vi "AudioTest.Config - Read Plot Analysis Params.vi"(11 "Config Dir":path=path "C:/MTE/Audio Test/Config") -> (1 "Avg(F)/Float(T)":bool, 2 "End Freq":dbl=20000.0, 3 "Start Freq":dbl=500.0)   [LabVIEW 2018]
uses:
  <vilib>/Utility/config.llb/Read Key (Boolean).vi
  <vilib>/Utility/config.llb/Write Key (Boolean).vi
  <vilib>/Utility/config.llb/Read Key (Double).vi
  <vilib>/Utility/config.llb/Write Key (Double).vi
  <vilib>/Utility/config.llb/NI_LVConfig.lvlib
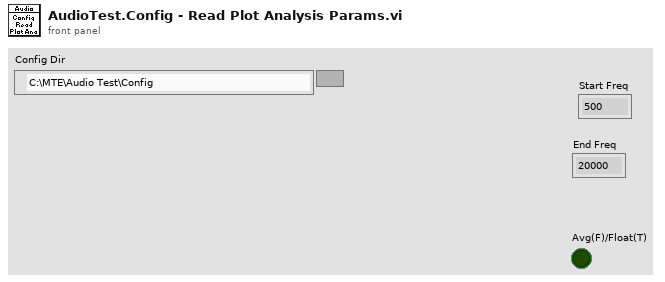
[diagram p1: front panel]
types:
  T1 = typedef "NI_LVConfig.lvlib/Config Data RefNum.ctl" = refnum<k1>
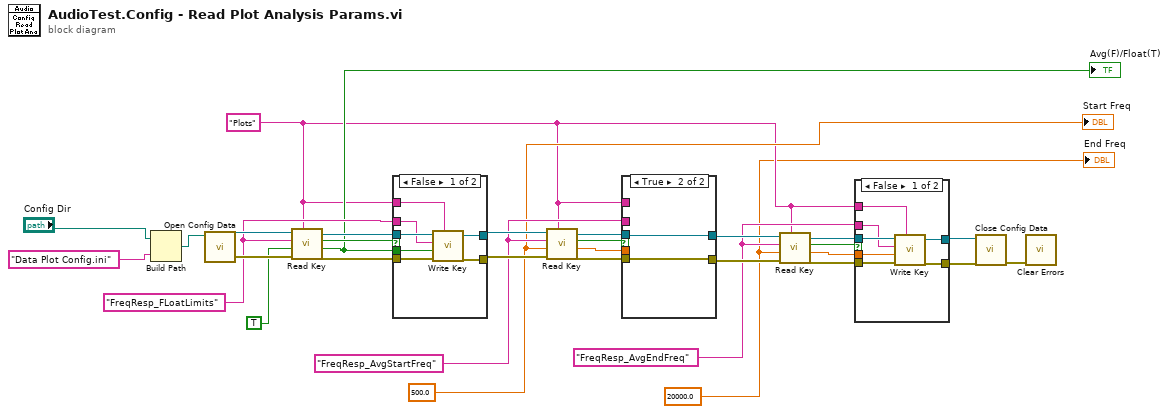
[diagram p0: block diagram]
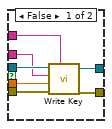
[diagram p3: hidden frame]
diagram:
  w6 = "FreqResp_AvgEndFreq" ("section")
  w2 = 20000.0 ("End Freq")
  w13 = 500.0 ("Start Freq")
  w14 = "FreqResp_AvgStartFreq" ("section")
  w26 = "FreqResp_FLoatLimits" ("section")
  w5 = "Plots" ("section")
  n1 = Build Path(base path="Config Dir", name or relative path="Data Plot Config.ini" ("Q Name")) -> (appended path=w29:path)
  n2 = call <vilib>:"Open Config Data.vi"("configuration file path"=w29) -> ("error out"=w30:errorcluster, "refnum"=w31:T1)  [unwired: 8 in, 1 out]
  n3 = call-poly <vilib>:"Read Key.vi"("section"=w5, "error in (no error)"=w30, "default value"=TRUE, "key"=w26, "refnum"=w31) -> ("error out"=w25:errorcluster, "value"=w22:bool, "found?"=w23:bool, "refnum out"=w27:T1)  [unwired: 3 in]
  "Avg(F)/Float(T)" <- w22
  n4 = case shown="False" w23 {
    tunnel: w27 -> [w38 w40]
    tunnel: w5 -> [w37 _]
    tunnel: w26 -> [w36 _]
    tunnel: w22 -> [w35 _]
    tunnel: w25 -> [w34 w39]
    tunnel: [w33 w39] -> w15
    tunnel: [w32 w40] -> w16
    frame False {
      n5 = call-poly <vilib>:"Write Key.vi"("section"=w37, "error in (no error)"=w34, "value"=w35, "key"=w36, "refnum"=w38) -> ("error out"=w33:errorcluster, "refnum out"=w32:T1)  [unwired: 4 in, 1 out]
    }
    frame True {
    }
  }
  n6 = call-poly <vilib>:"Read Key.vi"("section"=w5, "error in (no error)"=w15, "default value"=w13, "key"=w14, "refnum"=w16) -> ("error out"=w19:errorcluster, "value"=w21:dbl, "found?"=w20:bool, "refnum out"=w18:T1)  [unwired: 3 in]
  n7 = case shown="True" w20 {
    tunnel: w18 -> [w47 w49]
    tunnel: w5 -> [w46 _]
    tunnel: w14 -> [w45 _]
    tunnel: w21 -> [w44 _]
    tunnel: w19 -> [w43 w48]
    tunnel: [w42 w48] -> w8
    tunnel: [w41 w49] -> w7
    frame False {
      n8 = call-poly <vilib>:"Write Key.vi"("section"=w46, "error in (no error)"=w43, "value"=w44, "key"=w45, "refnum"=w47) -> ("error out"=w42:errorcluster, "refnum out"=w41:T1)  [unwired: 4 in, 1 out]
    }
    frame True {
    }
  }
  n9 = call-poly <vilib>:"Read Key.vi"("section"=w5, "error in (no error)"=w8, "default value"=w2, "key"=w6, "refnum"=w7) -> ("error out"=w11:errorcluster, "value"=w9:dbl, "found?"=w10:bool, "refnum out"=w12:T1)  [unwired: 3 in]
  n10 = case shown="False" w10 {
    tunnel: w12 -> [w56 w58]
    tunnel: w5 -> [w55 _]
    tunnel: w6 -> [w54 _]
    tunnel: w9 -> [w53 _]
    tunnel: w11 -> [w52 w57]
    tunnel: [w51 w57] -> w3
    tunnel: [w50 w58] -> w4
    frame False {
      n11 = call-poly <vilib>:"Write Key.vi"("section"=w55, "error in (no error)"=w52, "value"=w53, "key"=w54, "refnum"=w56) -> ("error out"=w51:errorcluster, "refnum out"=w50:T1)  [unwired: 4 in, 1 out]
    }
    frame True {
    }
  }
  n12 = call <vilib>:"Close Config Data.vi"("error in (no error)"=w3, "refnum"=w4) -> ("error out"=w24:errorcluster)  [unwired: 8 in, 1 out]
  n13 = call <vilib>:"Clear Errors.vi"("error in (no error)"=w24) -> ()  [unwired: 5 in, 2 out]
  "Start Freq" <- w13
  "End Freq" <- w2
